vi "hp83623a close.vi"(8 "error in (no error)":errorcluster, 11 "hp83623a Settings (in)":T1={"Frequency (Hz)"=0.0, "Power (dBm)"=0.0, "Enabled"=TRUE, "initialized"=FALSE, "RF Output On/Off"=TRUE, "External Trigger?"=FALSE, "VISA Session"="GPIB0::3::INSTR", "Generator Name"="Generator"}) -> (0 "error out":errorcluster)   [LabVIEW 2013, in "HP83623A_RF_Generator.lvclass"]
uses:
  HP83623A_RF_Generator.lvclass
  HP83623A.ctl
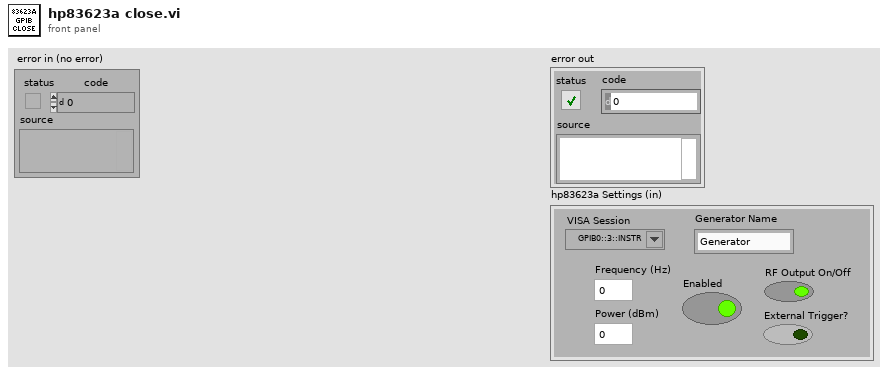
[diagram p1: front panel]
types:
  T1 = typedef "HP83623A_RF_Generator.lvclass/HP83623A.ctl" = cluster{"Frequency (Hz)":dbl, "Power (dBm)":dbl, "Enabled":bool, "initialized":bool, "RF Output On/Off":bool, "External Trigger?":bool, "VISA Session":refnum<visa-resource-name>, "Generator Name":string}
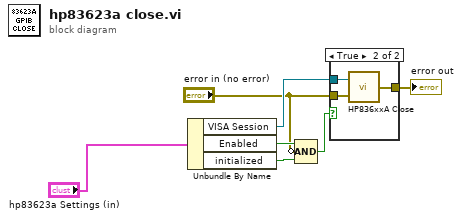
[diagram p0: block diagram]
diagram:
  n1 = Unbundle By Name("hp83623a Settings (in)") -> ("VISA Session"=w7:refnum<visa-resource-name>, "Enabled"=w5:bool, "initialized"=w3:bool)
  n2 = Compound Arithmetic op=AND(w5, invert "error in (no error)", w3) -> (w2:bool)
  n3 = case shown="True" w2 {
    tunnel: w7 -> [_ w11]
    tunnel: "error in (no error)" -> [w8 w10]
    tunnel: [w8 w9] -> w6
    frame False {
    }
    frame True {
      n4 = call "HP836xxA Close.vi"("error in (no error)"=w10, "VISA session"=w11) -> ("error out"=w9:errorcluster)
    }
  }
  "error out" <- w6
